vi "SVMDense_GridSearch_FromFile.vi"() -> ()   [LabVIEW 2015]
uses:
  LibSVM Sparse/Controls/Options Training.ctl
  LibSVM Sparse/Controls/Parameters C_SVC.ctl
  Tools/Controls/Binary_ConfusionMatrix.ctl
  <vilib>/Math Plots/3D Math Plots/3D Surface/3D Surface XCtrl/3D Surface.xctl
  LibSVM Sparse/Controls/Grid parameters.ctl
  LibSVM Sparse/Controls/Kernel.ctl
  LibSVM Sparse/Wrapper API/Controls/svm_kernel_type.ctl
  SubVIs/SVM Dense Train C_SVC.vi
  Tools/SubVIs/Dense - Scale Nodes Linear.vi
  Tools/SubVIs/Dense - Scale Problem Linear.vi
  Wrapper API/svmdense_train.vi
  Wrapper API/svmdense_predict.vi
panel:
  in  "Grid parameters":T1={"C start"=-5.0, "C end"=15.0, "C step"=4.0, "Gamma start"=-15.0, "Gamma end"=3.0, "Gamma step"=4.0, "K"=10, "random seed"=-1}
  out "Graph":refnum<class "3D Plot Datatype.lvclass">[](xcontrol)
  out "Gridsearch time (ms)":u32
  out "log2(gamma) max":dbl
  out "log2(C) max":dbl
  out "error out":errorcluster
  out "Binary Confusion Matrix":T2
  out "Misclassification counts":i32[](array[numeric])
  in  "libsvm":T5={"libsvm options"={"cache_size"=200.0, "eps"=0.001, "shrinking"=TRUE, "probability"=FALSE}, "libsvm weights"={"C"=1.0, "weight_label"=[], "weight"=[]}}
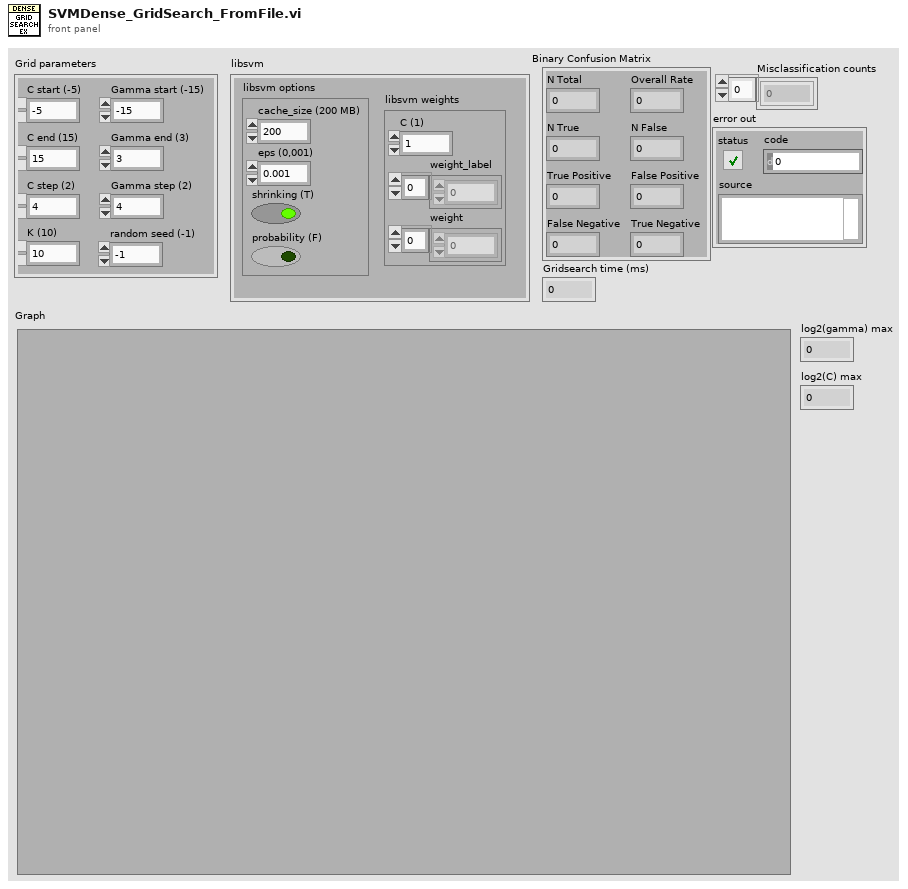
[diagram p1: front panel]
types:
  T1 = typedef "Grid parameters.ctl" = cluster{"C start":dbl, "C end":dbl, "C step":dbl, "Gamma start":dbl, "Gamma end":dbl, "Gamma step":dbl, "K":i32, "random seed":i32}
  T2 = typedef "Binary_ConfusionMatrix.ctl" = cluster{"N Total":u32, "N True":u32, "N False":u32, "Overall Rate":dbl, "True Positive":dbl, "False Positive":dbl, "False Negative":dbl, "True Negative":dbl}
  T3 = typedef "Options Training.ctl" = cluster{"cache_size":dbl, "eps":dbl, "shrinking":bool, "probability":bool}
  T4 = typedef "Parameters C_SVC.ctl" = cluster{"C":dbl, "weight_label":i32[], "weight":dbl[]}
  T5 = cluster{"libsvm options":T3, "libsvm weights":T4}
  T6 = typedef "svm_kernel_type.ctl" = enum32{"LINEAR", "POLY", "RBF", "SIGMOID", "PRECOMPUTED"}
  T7 = typedef "Kernel.ctl" = cluster{"Type":T6, "Degree":i32, "Gamma":dbl, "Coef0":dbl}
  T8 = typedef "svm_problem.ctl" = cluster{"y":dbl[], "x":cluster{T9[]}[]}
  T9 = typedef "svm_node.ctl" = cluster{"index":i32, "value":dbl}
  T10 = typedef "svmdense_problem.ctl" = cluster{"Y":dbl[], "X":cluster{"x":dbl[]}[]}
  T11 = typedef "svmdense_model.ctl" = cluster{"param":T12, "nr_class":i32, "l":i32, "SV":cluster{"Array":dbl[]}[], "sv_coef":dbl[][], "rho":dbl[], "probA":dbl[], "probB":dbl[], "sv_indices":i32[], "label":i32[], "nSV":i32[]}
  T12 = typedef "svm_parameter.ctl" = cluster{"svm_type":T13, "kernel_type":T6, "degree":i32, "gamma":dbl, "coef0":dbl, "cache_size":dbl, "eps":dbl, "C":dbl, "weight_label":i32[], "weight":dbl[], "nu":dbl, "p":dbl, "shrinking":bool, "probability":bool}
  T13 = typedef "svm_type.ctl" = enum32{"C_SVC", "NU_SVC", "ONE_CLASS", "EPSILON_SVR", "NU_SVR"}
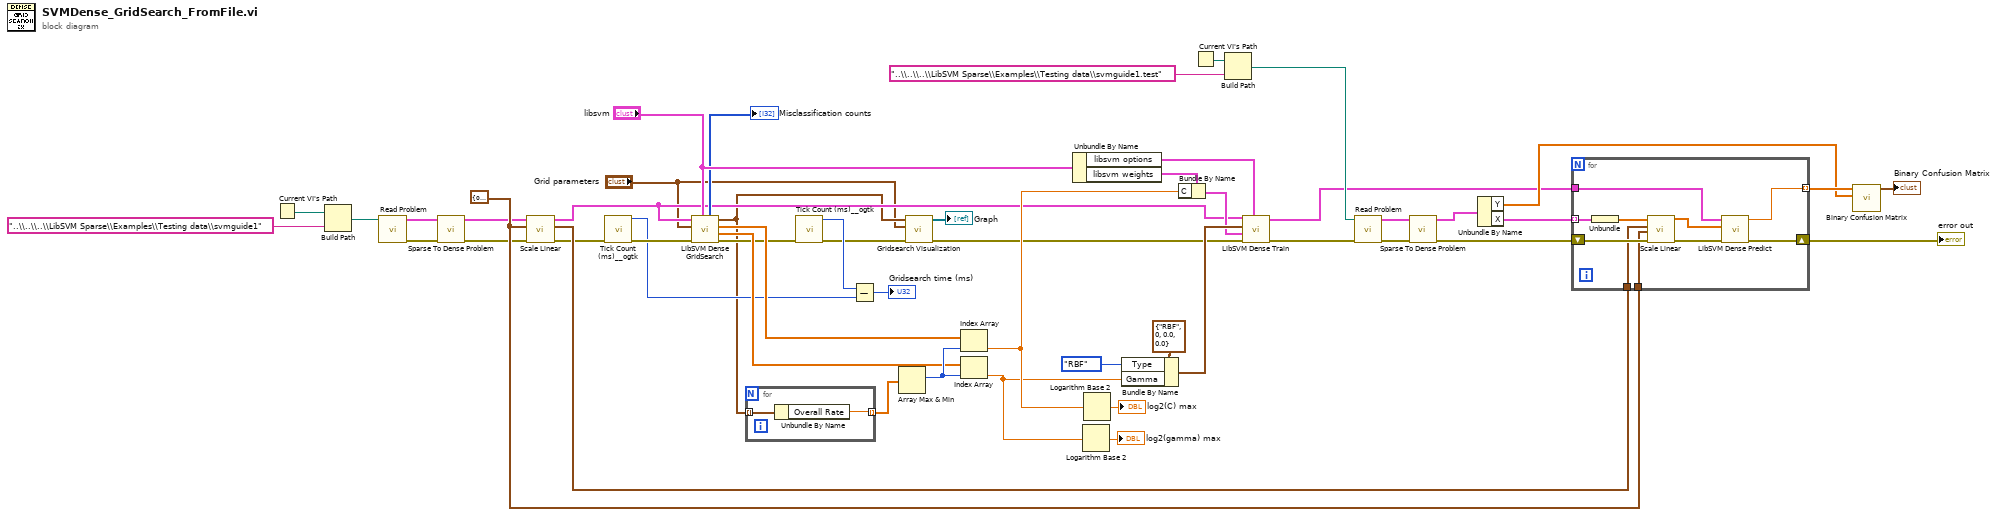
[diagram p0: block diagram]
diagram:
  w41 = cluster{"X lower":dbl, "X upper":dbl} {"X lower"=0.0, "X upper"=1.0} ("X Scaling limits")
  n1 = Current VI's Path() -> (path=w51:path)
  n2 = Build Path(base path=w51, name or relative path="..\\..\\..\\LibSVM Sparse\\Examples\\Testing data\\svmguide1") -> (appended path=w15:path)
  n3 = call "Read Problem.vi"("file path (use dialog)"=w15) -> ("error out"=w31:errorcluster, "svm_problem"=w32:T8)  [unwired: 9 in]
  n4 = call "Sparse To Dense Problem.vi"("error in (no error)"=w31, "Sparse Problem"=w32) -> ("error out"=w30:errorcluster, "Dense Problem"=w29:T10)  [unwired: 8 in]
  n5 = call-poly "Scale Linear.vi"("error in (no error)"=w30, "X Scaling limits"=w41, "Problem"=w29) -> ("error out"=w12:errorcluster, "xmaxmin"=w42:cluster{"min":dbl, "max":dbl}[], "Scaled problem"=w9:T10)  [unwired: 6 in]
  n6 = call <userlib>:"Tick Count (ms)__ogtk.vi"("error in (no error)"=w12) -> ("error out"=w11:errorcluster, "millisecond timer value"=w7:u32)  [unwired: 9 in]
  n7 = call "LibSVM Dense GridSearch.vi"("libsvm"="libsvm", "error in (no error)"=w11, "Grid parameters"="Grid parameters", "Problem"=w9) -> ("error out"=w10:errorcluster, "gamma"=w26:dbl[], "C"=w25:dbl[], "Confusion matrices"=w2:T2[], "Misclassification counts"=→"Misclassification counts":i32[])  [unwired: 3 in]
  n8 = for {
    tunnel: w2 -> [w53] mode=indexing
    tunnel: [w52] -> w50 mode=indexing
    n9 = Unbundle By Name(w53) -> ("Overall Rate"=w52:dbl)
  }
  n10 = call <userlib>:"Tick Count (ms)__ogtk.vi"("error in (no error)"=w10) -> ("error out"=w4:errorcluster, "millisecond timer value"=w8:u32)  [unwired: 9 in]
  n11 = Subtract(x=w8, y=w7) -> (x-y=→"Gridsearch time (ms)":u32)
  n12 = Array Max & Min(array=w50) -> (max index (indices)=w49:i32)  [unwired: 3 out]
  n13 = call "Gridsearch Visualization.vi"("error in (no error)"=w4, "Grid parameters"="Grid parameters", "Confusion matrices"=w2) -> ("error out"=w3:errorcluster, "3D Surface Plot"=→"Graph":refnum<class "3D Plot Datatype.lvclass">[])  [unwired: 7 in]
  n14 = Index Array(array=w25, index=w49) -> (element=w36:dbl)
  n15 = Index Array(array=w26, index=w49) -> (element=w35:dbl)
  n16 = Unbundle By Name("libsvm") -> ("libsvm options"=w21:T3, "libsvm weights"=w48:T4)
  n17 = Logarithm Base 2(1:w35) -> (0:→"log2(gamma) max":dbl)
  n18 = Logarithm Base 2(1:w36) -> (0:→"log2(C) max":dbl)
  n19 = Bundle By Name(cluster=T7 {"Type"=enum."RBF", "Degree"=0, "Gamma"=0.0, "Coef0"=0.0} ("Kernel"), "Type"=svm_kernel_type."RBF", "Gamma"=w35) -> (w23:T7)
  n20 = Bundle By Name(cluster=w48, "C"=w36) -> (w22:T4)
  n21 = Current VI's Path() -> (path=w45:path)
  n22 = Build Path(base path=w45, name or relative path="..\\..\\..\\LibSVM Sparse\\Examples\\Testing data\\svmguide1.test") -> (appended path=w44:path)
  n23 = call-poly "LibSVM Dense Train.vi"("Options"=w21, "error in (no error)"=w3, "Param C_SVC"=w22, "Kernel"=w23, "Dense problem"=w9) -> ("error out"=w20:errorcluster, "Model"=w24:T11)  [unwired: 5 in]
  n24 = call "Read Problem.vi"("error in (no error)"=w20, "file path (use dialog)"=w44) -> ("error out"=w18:errorcluster, "svm_problem"=w19:T8)  [unwired: 8 in]
  n25 = call "Sparse To Dense Problem.vi"("error in (no error)"=w18, "Sparse Problem"=w19) -> ("error out"=w16:errorcluster, "Dense Problem"=w17:T10)  [unwired: 8 in]
  n26 = Unbundle By Name(w17) -> ("Y"=w39:dbl[], "X"=w43:cluster{"x":dbl[]}[])
  n27 = for {
    tunnel: w43 -> [w63] mode=indexing
    tunnel: w42 -> [w60]
    tunnel: w41 -> [w59]
    tunnel: w24 -> [w58]
    shift-right: [w55] -> w37
    shift-left: w16 -> [w61]
    tunnel: [w54] -> w40 mode=indexing
    n28 = Unbundle(w63) -> ("x"=w62:dbl[])
    n29 = call-poly "Scale Linear.vi"("error in (no error)"=w61, "Scaling limits"=w59, "xmaxmin"=w60, "x"=w62) -> ("error out"=w56:errorcluster, "x scaled"=w57:dbl[])  [unwired: 6 in]
    n30 = call-poly "LibSVM Dense Predict.vi"("error in (no error)"=w56, "x"=w57, "Model"=w58) -> ("error out"=w55:errorcluster, "Predicted label"=w54:dbl)  [unwired: 7 in]
  }
  "error out" <- w37
  n31 = call "Binary Confusion Matrix.vi"("Actual Labels"=w39, "Predicted Labels"=w40) -> ("Binary Confusion Matrix"=→"Binary Confusion Matrix":T2)  [unwired: 9 in]
